vi "Build Report File Path.vi"(8 "error in (no error)":errorcluster, 11 "File Path in":path) -> (0 "error out":errorcluster, 3 "Report Path out":path)   [LabVIEW 2018]
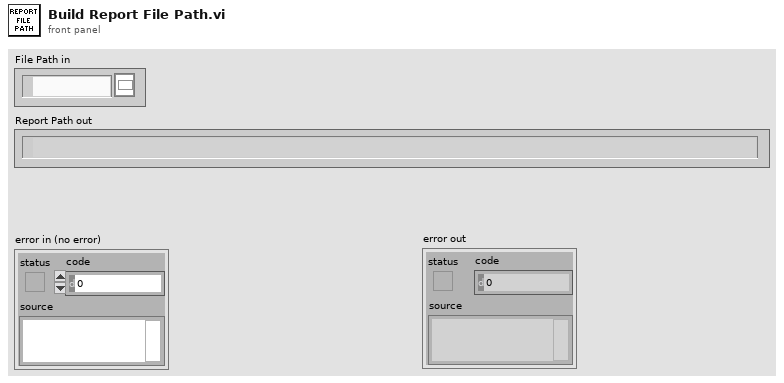
[diagram p1: front panel]
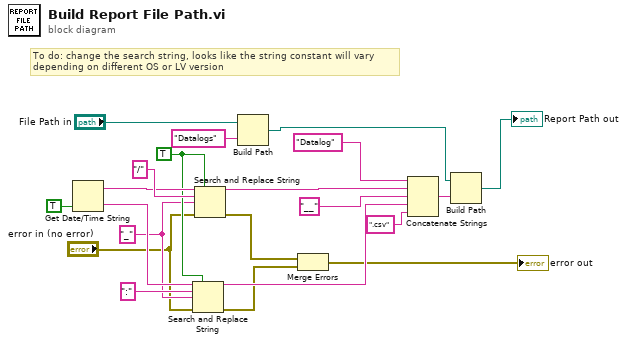
[diagram p0: block diagram]
diagram:
  w9 = TRUE ("replace all? (F)")
  w8 = "_" ("replace string (\"\")")
  # "To do: change the search string, looks like the string constant will vary\ndepending on different OS or LV version"
  n1 = Get Date/Time String(want seconds? (F)=TRUE) -> (date string=w19:string, time string=w18:string)  [unwired: 2 in]
  n2 = Search and Replace String(replace all?=w9, input string=w18, search string=":", replace string=w8, error in="error in (no error)") -> (result string=w14:string, error out=w5:errorcluster)  [unwired: 3 in, 2 out]
  n3 = Search and Replace String(replace all?=w9, input string=w19, search string="/", replace string=w8, error in="error in (no error)") -> (result string=w16:string, error out=w6:errorcluster)  [unwired: 3 in, 2 out]
  n4 = Build Path(base path="File Path in", name or relative path="Datalogs") -> (appended path=w1:path)
  n5 = Merge Errors(w6, w5) -> (→"error out":errorcluster)
  n6 = Concatenate Strings("Datalog" ("string"), w16, "__" ("string"), w14, ".csv" ("string")) -> (w12:string)
  n7 = Build Path(base path=w1, name or relative path=w12) -> (appended path=→"Report Path out":path)
